vi "ShuffleArray.vi"(7 "Monochromator in":T1={"Type"=enum."Oriel", "Wavelength (nm)"=0.25, "Grating, gr/mm"=enum."1200", "Grating mode"=enum."IR", "Spectrum mode"={"Spectrum mode?"=FALSE, "Start wavelength (nm)"=0.0, "End wavelength (nm)"=0.0, "Wavelength step (nm)"=0.0, "Wavelength array"=[], "array index"=0}, "PTI"={"Delay before read (ms)"=1000, "Mono 1"={"Timeout (ms)"=1000, "Resource Name"="COM1", "Baud Rate"=9600, "Data Bits"=8, "Parity"=0, "Stop Bits"=10, "Flow Control"=0}, "Mono 2"={"Timeout (ms)"=1000, "Resource Name"="COM1", "Baud Rate"=9600, "Data Bits"=8, "Parity"=0, "Stop Bits"=10, "Flow Control"=0}, "Two PTI Monochromators?"=FALSE}, "Oriel (custom)"={"reference"=refnum}, "Force wavelength confirmation (PTI)?"=FALSE} {"PTI"."Mono 2"."Flow Control" items=["1.0"=10, "1.5"=15, "2.0"=20]; "PTI"."Mono 2"."Stop Bits" items=["None", "Odd", "Even", "Mark", "Space"]; "PTI"."Mono 2"."Parity" items=["None", "Odd", "Even", "Mark", "Space"]; "PTI"."Mono 1"."Flow Control" items=["1.0"=10, "1.5"=15, "2.0"=20]; "PTI"."Mono 1"."Stop Bits" items=["None", "Odd", "Even", "Mark", "Space"]; "PTI"."Mono 1"."Parity" items=["None", "Odd", "Even", "Mark", "Space"]}, 8 "Error In":errorcluster) -> (0 "Error Out":errorcluster, 5 "Monochromator out":T1={"Type"=enum."Oriel", "Wavelength (nm)"=0.25, "Grating, gr/mm"=enum."1200", "Grating mode"=enum."IR", "Spectrum mode"={"Spectrum mode?"=FALSE, "Start wavelength (nm)"=0.0, "End wavelength (nm)"=0.0, "Wavelength step (nm)"=0.0, "Wavelength array"=[], "array index"=0}, "PTI"={"Delay before read (ms)"=1000, "Mono 1"={"Timeout (ms)"=1000, "Resource Name"="COM1", "Baud Rate"=9600, "Data Bits"=8, "Parity"=0, "Stop Bits"=10, "Flow Control"=0}, "Mono 2"={"Timeout (ms)"=1000, "Resource Name"="COM1", "Baud Rate"=9600, "Data Bits"=8, "Parity"=0, "Stop Bits"=10, "Flow Control"=0}, "Two PTI Monochromators?"=FALSE}, "Oriel (custom)"={"reference"=refnum}, "Force wavelength confirmation (PTI)?"=FALSE} {"PTI"."Mono 2"."Flow Control" items=["1.0"=10, "1.5"=15, "2.0"=20]; "PTI"."Mono 2"."Stop Bits" items=["None", "Odd", "Even", "Mark", "Space"]; "PTI"."Mono 2"."Parity" items=["None", "Odd", "Even", "Mark", "Space"]; "PTI"."Mono 1"."Flow Control" items=["1.0"=10, "1.5"=15, "2.0"=20]; "PTI"."Mono 1"."Stop Bits" items=["None", "Odd", "Even", "Mark", "Space"]; "PTI"."Mono 1"."Parity" items=["None", "Odd", "Even", "Mark", "Space"]})   [LabVIEW 2017, in "Monochromator.lvlib"]
uses:
  Monochromator.lvlib
  Controls/Params.ctl
  Controls/Type.ctl
  Controls/GratingValues.ctl
  Controls/Grating.ctl
  PTI/Controls/Params.ctl
  Controls/VISA parameters.ctl
  Custom Oriel drivers/Controls/Params.ctl
  C:/Project Work/icl-optical-software-rewrite/Optical Software Code Simplified/Modules/Monochromator/Cornerstone.dll
  Cornerstone.dll
  4324117d-80fa-4d98-9588-6f8792818a0f.vi
  Serial comms/Serial comms.lvlib
  PTI/PTI.lvlib
  Custom Oriel drivers/Oriel (custom drivers).lvlib
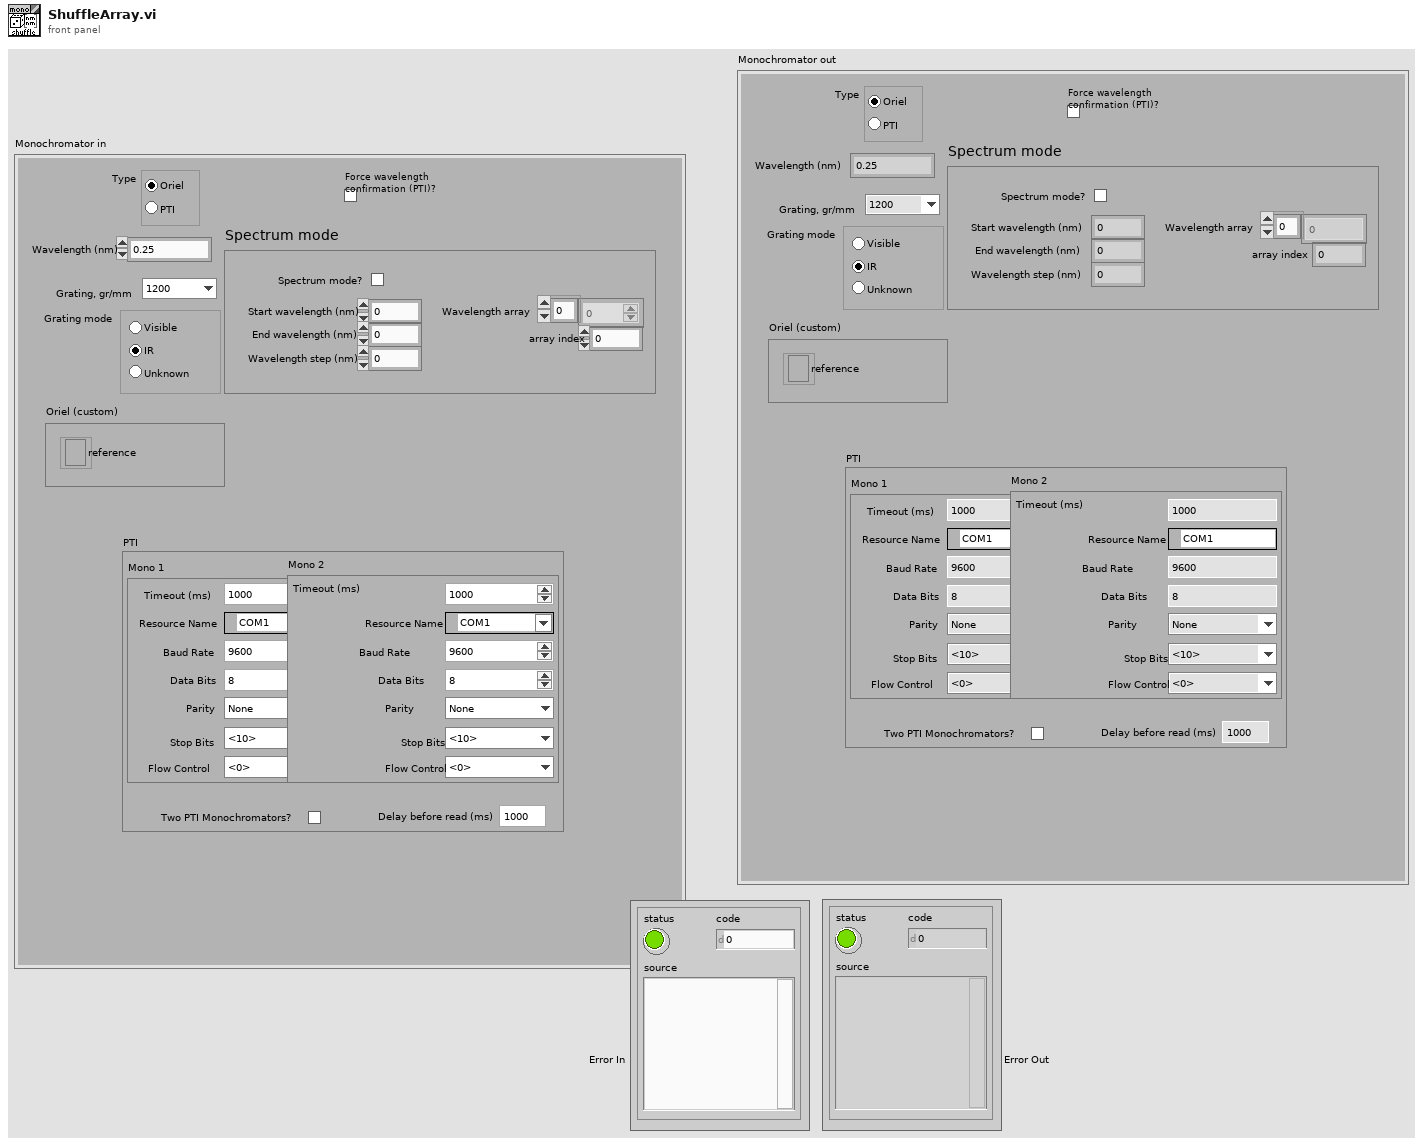
[diagram p1: front panel]
types:
  T1 = typedef "Monochromator.lvlib/Params.ctl" = cluster{"Type":T2, "Wavelength (nm)":dbl, "Grating, gr/mm":T3, "Grating mode":T4, "Spectrum mode":cluster{"Spectrum mode?":bool, "Start wavelength (nm)":dbl, "End wavelength (nm)":dbl, "Wavelength step (nm)":dbl, "Wavelength array":dbl[], "array index":u32}, "PTI":T5, "Oriel (custom)":T7, "Force wavelength confirmation (PTI)?":bool}
  T2 = typedef "Monochromator.lvlib/Type.ctl" = enum32{"Oriel", "PTI"}
  T3 = typedef "Monochromator.lvlib/GratingValues.ctl" = enum16{"2400", "1800", "1200", "600", "300", "150"}
  T4 = typedef "Monochromator.lvlib/Grating.ctl" = enum32{"Unknown", "Visible", "IR"}
  T5 = typedef "Monochromator.lvlib/PTI.lvlib/Params.ctl" = cluster{"Delay before read (ms)":u32, "Mono 1":T6, "Mono 2":T6, "Two PTI Monochromators?":bool}
  T6 = typedef "Serial comms.lvlib/VISA parameters.ctl" = cluster{"Timeout (ms)":u32, "Resource Name":refnum<visa-resource-name>, "Baud Rate":u32, "Data Bits":u16, "Parity":u16, "Stop Bits":u16, "Flow Control":u16}
  T7 = typedef "Monochromator.lvlib/Oriel (custom drivers).lvlib/Params.ctl" = cluster{"reference":refnum<k24>}
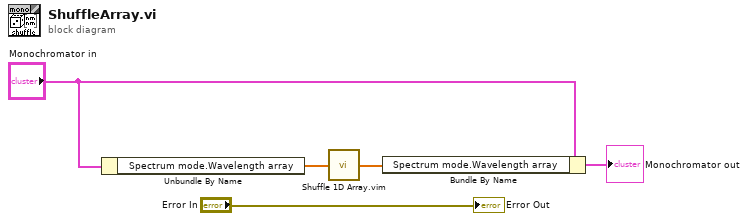
[diagram p0: block diagram]
diagram:
  n1 = Unbundle By Name("Monochromator in") -> ("Spectrum mode.Wavelength array"=w5:dbl[])
  n2 = call "Shuffle 1D Array.vim"("array"=w5) -> ("shuffled array"=w4:dbl[])  [unwired: 4 in]
  n3 = Bundle By Name(cluster="Monochromator in", "Spectrum mode.Wavelength array"=w4) -> (→"Monochromator out":T1)
  "Error Out" <- "Error In"
